vi "panel_update_status_string.vi"(8 "error in (no error)":errorcluster, 10 "String":string, 11 "hydraharp_panel in":refnum<class "picoharp_panel.lvclass">) -> (0 "error out":errorcluster, 3 "hydraharp_panel out":refnum<class "picoharp_panel.lvclass">)   [LabVIEW 2015, in "picoharp_panel.lvclass"]
uses:
  picoharp_panel.lvclass
  picoharp_panel.lvclass/picoharp_panel.ctl
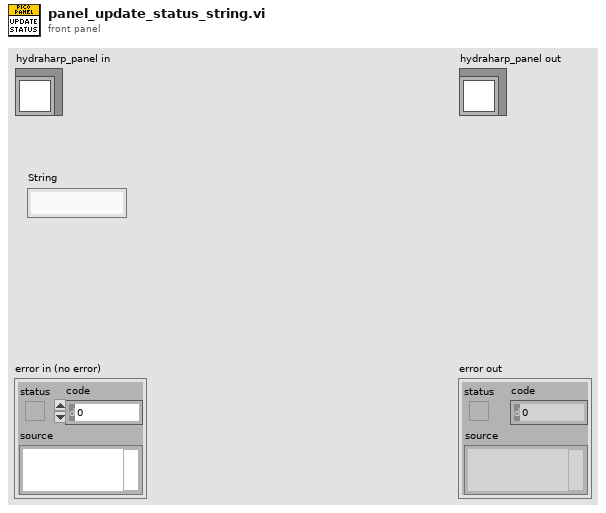
[diagram p1: front panel]
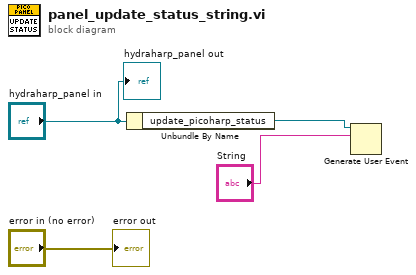
[diagram p0: block diagram]
diagram:
  n1 = Unbundle By Name("hydraharp_panel in") -> ("update_picoharp_status"=w2:refnum<user-event>)
  n2 = Generate User Event(user event=w2, event data cluster="String") -> ()  [unwired: 2 in, 2 out]
  "error out" <- "error in (no error)"
  "hydraharp_panel out" <- "hydraharp_panel in"
